vi "GetOneStepIndex.vi"(8 "error in (no error)":errorcluster) -> (0 "error out":errorcluster, 2 "OneStep?":bool, 3 "OneStepIndex":u32)   [LabVIEW 2016, in "SeqProcessor.lvlib"]
uses:
  SeqProcessor.lvlib
  <vilib>/addons/PointValueMap/subVIs/Point_Read_variant.vi
  <vilib>/addons/PointValueMap/PointValueMap.lvlib
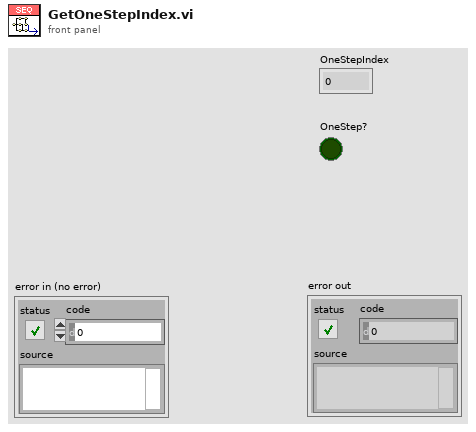
[diagram p1: front panel]
types:
  T1 = typedef "PointValueMap.lvlib/PointMap.ctl" = refnum<data-value>
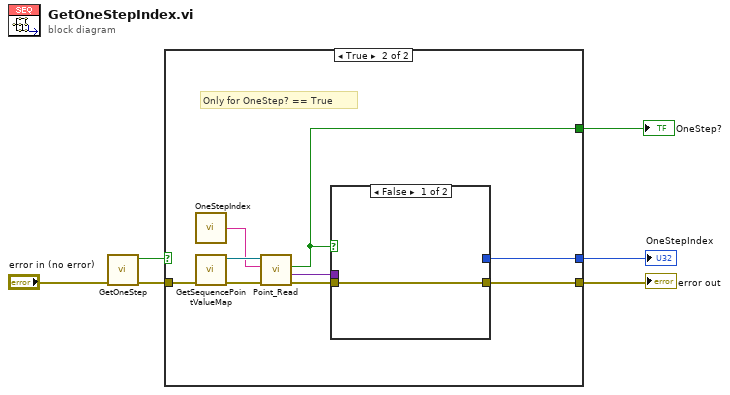
[diagram p0: block diagram]
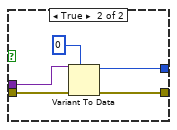
[diagram p3: hidden frame]
diagram:
  n1 = call "GetOneStep.vi"("error in (no error)"="error in (no error)") -> ("error out"=w5:errorcluster, "OneStep?"=w4:bool)  [unwired: 8 in, 1 out]
  n2 = case shown="True" w4 {
    tunnel: w5 -> [w7 w12]
    tunnel: [w7 w10] -> w3
    tunnel: [_ w9] -> w2
    tunnel: [_ w8] -> w1
    frame False {
    }
    frame True {
      # "Only for OneStep? == True"
      n3 = call "OneStepIndex.vi"() -> ("OneStepIndex"=w11:string)  [unwired: 5 in]
      n4 = call "GetSequencePointValueMap.vi"("error in (no error)"=w12) -> ("error out"=w14:errorcluster, "SeqMap"=w13:T1)  [unwired: 9 in]
      n5 = call-poly <vilib>:"Point_Read.vi"("Error In"=w14, "Tag"=w11, "Map"=w13) -> ("Error Out"=w16:errorcluster, "Value"=w15:variant, "Found?"=w9:bool)  [unwired: 3 in, 3 out]
      n6 = case shown="False" w9 {
        tunnel: w16 -> [w17 w22]
        tunnel: [w17 w21] -> w10
        tunnel: w15 -> [_ w20]
        tunnel: [_ w18] -> w8
        frame False {
        }
        frame True {
          n7 = Variant To Data(error in=w22, type=u32 0, Variant=w20) -> (data=w18:u32, error out=w21:errorcluster)
        }
      }
    }
  }
  "error out" <- w3
  "OneStep?" <- w2
  "OneStepIndex" <- w1
